vi "Reset Window.vi"(8 "error in (no error)":errorcluster, 11 "Rigol DG822 Square in":refnum<class "Rigol DG822 Square.lvclass">) -> (0 "error out":errorcluster, 3 "Rigol DG822 Square out":refnum<class "Rigol DG822 Square.lvclass">)   [LabVIEW 2021, in "Rigol DG822 UI.lvlib" / "Rigol DG822 Square.lvlib" / "Rigol DG822 Square.lvclass"]
uses:
  Rigol DG822 Square.lvclass
  General/Files/lvlibp/Actors.lvlibp/Actors/Actors/Actors.lvclass
  D:/LabVIEW/General/Files/lvlibp/Actors.lvlibp/Actors/Actors/Actors.lvclass
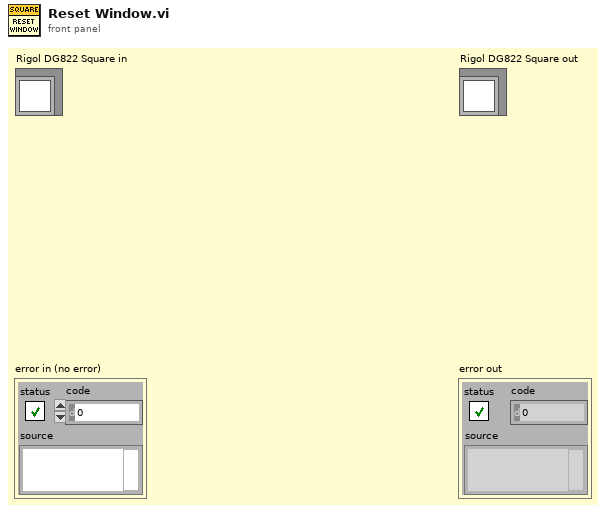
[diagram p1: front panel]
types:
  T1 = cluster{"Control Label 5":string, "Control Label 6":string, "Control Label":string, "Control Label 2":string, "Control Label 3":string, "Control Label 4":string}
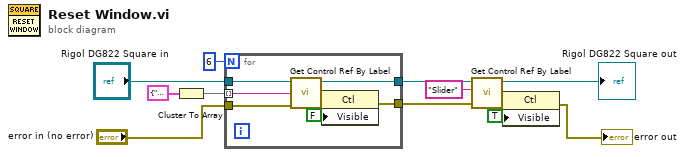
[diagram p0: block diagram]
diagram:
  n1 = Cluster To Array(cluster=T1 {"Control Label 5"="FreqUnit", "Control Label 6"="PeriodUnit", "Control Label"="AmplUnit", "Control Label 2"="HighLUnit", "Control Label 3"="OffsetUnit", "Control Label 4"="LowLUnit"}) -> (array=w7:string[])
  n2 = for {
    N: 6 -> [_]
    tunnel: [w18] -> w3
    tunnel: "Rigol DG822 Square in" -> [w17]
    tunnel: w7 -> [w16] mode=indexing
    tunnel: "error in (no error)" -> [w15]
    tunnel: [w14] -> w1
    n3 = call "Get Control Ref By Label.vi"("error in (no error)"=w15, "Control Label"=w16, "Actors in"=w17) -> ("error out"=w20:errorcluster, "Control Ref"=w19:refnum<vi>, "Actors out"=w18:refnum<class "Rigol DG822 Square.lvclass">)  [unwired: 6 in]
    n4 = property class="Ctl"(reference=w19, error in=w20, "Visible"=FALSE) -> (error out=w14:errorcluster)  [unwired: 1 out]
  }
  n5 = call "Get Control Ref By Label.vi"("error in (no error)"=w1, "Control Label"="Slider", "Actors in"=w3) -> ("error out"=w11:errorcluster, "Control Ref"=w10:refnum<vi>, "Actors out"=→"Rigol DG822 Square out":refnum<class "Rigol DG822 Square.lvclass">)  [unwired: 6 in]
  n6 = property class="Ctl"(reference=w10, error in=w11, "Visible"=TRUE) -> (error out=→"error out":errorcluster)  [unwired: 1 out]
